vi "Matches.vi"(8 "error in (no error)":errorcluster, 10 "Actual":variant, 11 "StringContains in":refnum<class "StringContains.lvclass">) -> (0 "error out":errorcluster, 2 "Result":bool, 3 "StringContains out":refnum<class "StringContains.lvclass">)   [LabVIEW 2019, in "Constraint.lvlib" / "StringContains.lvclass"]
doc: "Evaluates the constraint for <B>Actual</B>. Returns true if the constraint is met."
uses:
  StringContains.lvclass
  StringContains.lvclass/StringContains.ctl
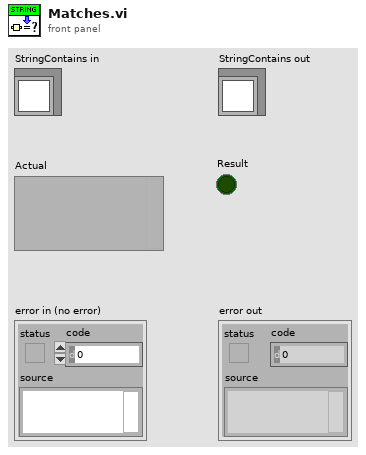
[diagram p1: front panel]
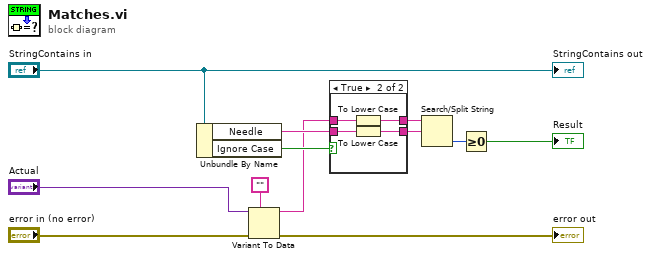
[diagram p0: block diagram]
diagram:
  n1 = Unbundle By Name("StringContains in") -> ("Needle"=w4:string, "Ignore Case"=w5:bool)
  n2 = Variant To Data(error in="error in (no error)", type="", Variant="Actual") -> (data=w2:string, error out=→"error out":errorcluster)
  n3 = case shown="True" w5 {
    tunnel: w4 -> [w14 w17]
    tunnel: [w14 w15] -> w3
    tunnel: w2 -> [w13 w18]
    tunnel: [w13 w16] -> w1
    frame False {
    }
    frame True {
      n4 = To Lower Case(string=w18) -> (all lower case string=w16:string)
      n5 = To Lower Case(string=w17) -> (all lower case string=w15:string)
    }
  }
  n6 = Search/Split String(string=w1, search string/char (-)=w3) -> (offset of match=w7:i32)  [unwired: 1 in, 2 out]
  n7 = Greater Or Equal To 0?(x=w7) -> (x >= 0?=→"Result":bool)
  "StringContains out" <- "StringContains in"
